vi "Array of Double_Write Index.vi"(9 "Value":dbl[](array[numeric]), 11 "Index":i32) -> ()   [LabVIEW 2016, in "CVT.lvlib" / "Current Value Table.lvlib"]
doc: "This VI takes a memory index (I32) and will perform a write on that index. This VI has no error handling for increased performance. If the index is invalid, no data will be transferred."
uses:
  Current Value Table.lvlib
  Type Defs/Memory Commands.ctl
  Array of Double_Memory Block.vi
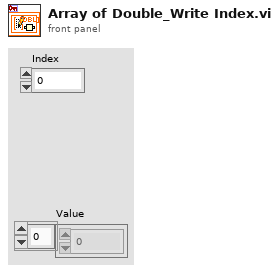
[diagram p1: front panel]
types:
  T1 = typedef "CVT.lvlib/Current Value Table.lvlib/Memory Commands.ctl" = enum16{"Init", "Add Data", "Read", "Read Group", "Read All", "Write", "Write Group", "Get Size"}
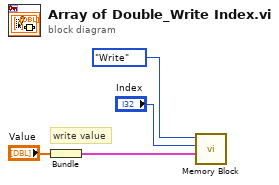
[diagram p0: block diagram]
diagram:
  # "write value"
  n1 = Bundle("Value"="Value") -> (w1:cluster{"Value":dbl[]})  [unwired: 1 in]
  n2 = call-poly "Memory Block.vi"("Value"=w1, "Index"="Index", "Method"=Memory_Commands."Write") -> ()  [unwired: 6 in, 3 out]
